vi "SQL_6220_data_insert.vi"(0 "数据":T1={"时间"=timestamp(3515985789.500352 s since 1904-01-01), "陪试轴承润滑单元出油温度1"=array[32000 elements], "陪试轴承润滑单元出油温度2"=array[32000 elements], "轴承外圈温度"=array[32000 elements], "出油温度"=array[32000 elements], "摩擦力1"=array[32000 elements], "摩擦力2"=array[32000 elements], "径向油缸力"=array[80000 elements], "轴向油缸力"=array[80000 elements], "转速"=array[80000 elements]}) -> (7 "error out":errorcluster, 8 "数据插入时间ms":u32)   [LabVIEW 2014]
uses:
  <vilib>/addons/database/Connection.llb/DB Tools Open Connec (String).vi
  <vilib>/addons/database/Connection.llb/Conn Execute.vi
  <vilib>/addons/database/Recordset.llb/Rec Destroy - Connection.vi
  <vilib>/addons/database/NI_Database_API.lvlib
panel:
  out "x-y":u32
  out "毫秒计时值 2":u32
  out "毫秒计时值":u32
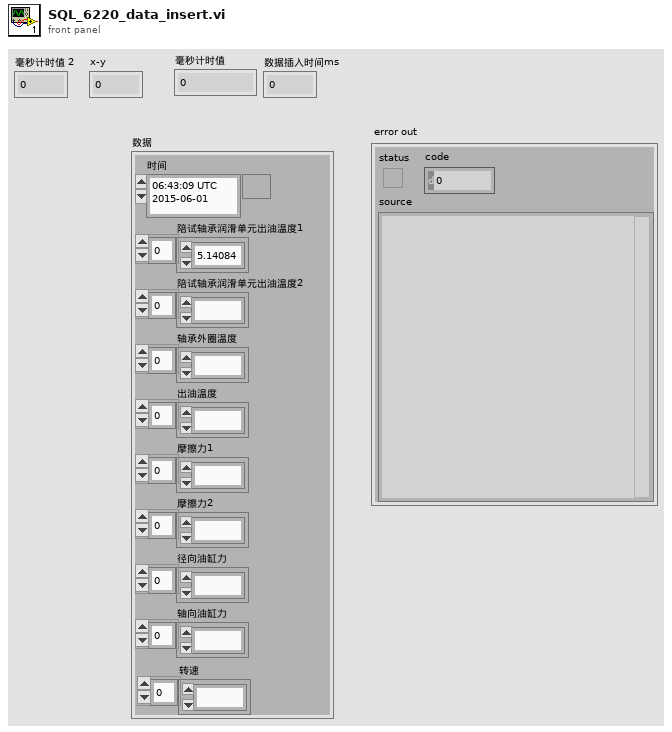
[diagram p1: front panel]
types:
  T1 = cluster{"时间":timestamp, "陪试轴承润滑单元出油温度1":sgl[], "陪试轴承润滑单元出油温度2":sgl[], "轴承外圈温度":sgl[], "出油温度":sgl[], "摩擦力1":sgl[], "摩擦力2":sgl[], "径向油缸力":sgl[], "轴向油缸力":sgl[], "转速":sgl[]}
  T2 = cluster{string, string, string, string, string, string, string, string, string}
  T3 = typedef "NI_Database_API.lvlib/Conn ObjectReference.ctl" = refnum<k1>
  T4 = typedef "NI_Database_API.lvlib/Rec ObjectReference.ctl" = refnum<k1>
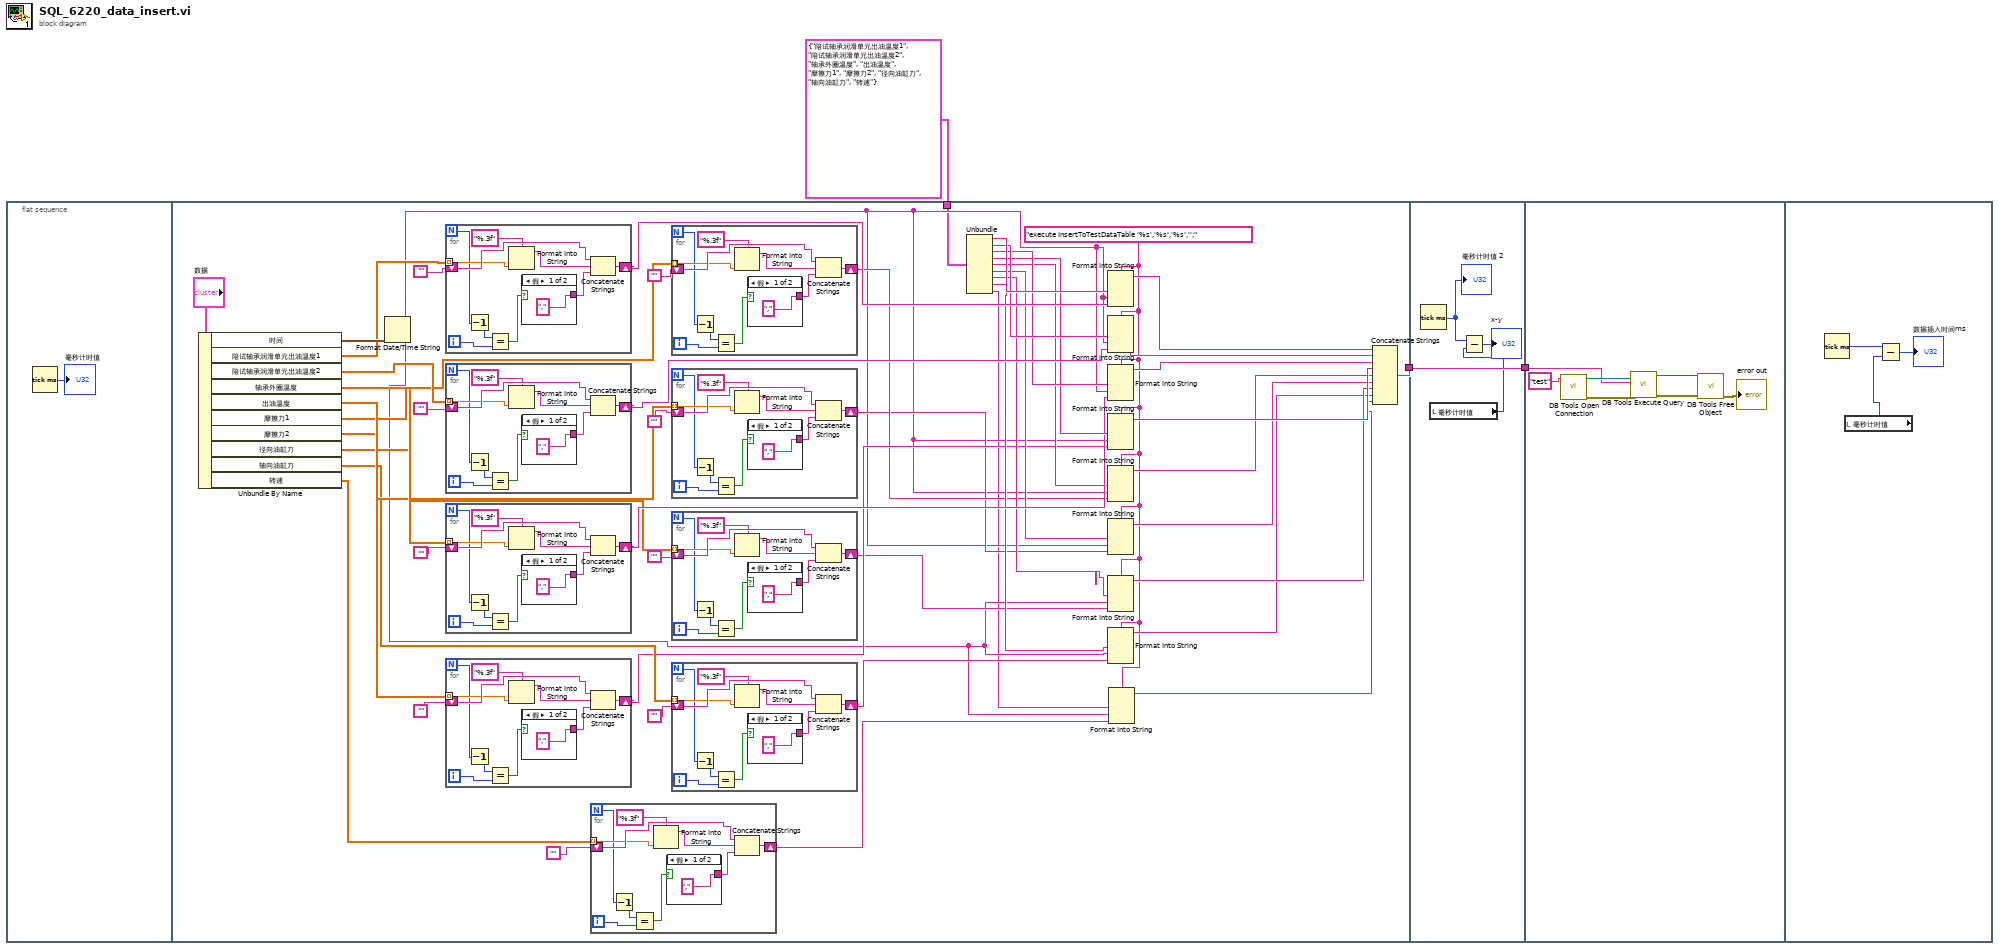
[diagram p0: block diagram]
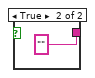
[diagram p2: hidden frame]
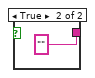
[diagram p3: hidden frame]
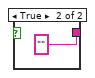
[diagram p4: hidden frame]
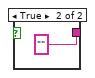
[diagram p5: hidden frame]
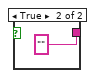
[diagram p6: hidden frame]
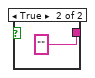
[diagram p7: hidden frame]
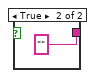
[diagram p8: hidden frame]
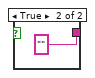
[diagram p9: hidden frame]
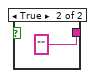
[diagram p10: hidden frame]
diagram:
  n1 = flat-sequence {
    tunnel: [w55] -> w3
    tunnel: T2 {"陪试轴承润滑单元出油温度1", "陪试轴承润滑单元出油温度2", "轴承外圈温度", "出油温度", "摩擦力1", "摩擦力2", "径向油缸力", "轴向油缸力", "转速"} ("通道名") -> [w5]
    tunnel: w3 -> [w167]
    tunnel: [w167] -> w2
    tunnel: w2 -> [w168]
    frame #0 {
      n2 = Tick Count (ms)() -> (millisecond timer value=→"毫秒计时值":u32)
    }
    frame #1 {
      w7 = "execute InsertToTestDataTable '%s','%s','%s','';"
      n3 = Unbundle By Name("数据") -> ("时间"=w54:timestamp, "陪试轴承润滑单元出油温度1"=w49:sgl[], "陪试轴承润滑单元出油温度2"=w48:sgl[], "轴承外圈温度"=w46:sgl[], "出油温度"=w44:sgl[], "摩擦力1"=w33:sgl[], "摩擦力2"=w32:sgl[], "径向油缸力"=w31:sgl[], "轴向油缸力"=w30:sgl[], "转速"=w12:sgl[])
      n4 = Format Date/Time String(seconds (now)=w54) -> (date/time string=w9:string)  [unwired: 2 in]
      n5 = for "For循环" {
        N -> [w154]
        tunnel: w49 -> [w159] mode=indexing
        shift-right: [w160] -> w51
        shift-left: "" -> [w161]
        i -> [w156]
        n6 = Decrement(x=w154) -> (x-1=w155:i32)
        n7 = Equal?(x=w155, y=w156) -> (x = y?=w153:bool)
        n8 = Format Into String(format string="%.3f", w159) -> (resulting string=w158:string)  [unwired: 2 in, 1 out]
        n9 = case shown="假" w153 {
          tunnel: ["," ""] -> w152
          frame False {
          }
          frame True {
          }
        }
        n10 = Concatenate Strings(w161, w158, w152) -> (w160:string)
      }
      n11 = for "For循环" {
        N -> [w142]
        tunnel: w48 -> [w147] mode=indexing
        shift-right: [w148] -> w42
        shift-left: "" -> [w149]
        i -> [w144]
        n12 = Decrement(x=w142) -> (x-1=w143:i32)
        n13 = Equal?(x=w143, y=w144) -> (x = y?=w141:bool)
        n14 = Format Into String(format string="%.3f", w147) -> (resulting string=w146:string)  [unwired: 2 in, 1 out]
        n15 = case shown="假" w141 {
          tunnel: ["," ""] -> w140
          frame False {
          }
          frame True {
          }
        }
        n16 = Concatenate Strings(w149, w146, w140) -> (w148:string)
      }
      n17 = for "For循环" {
        N -> [w130]
        tunnel: w46 -> [w135] mode=indexing
        shift-right: [w136] -> w37
        shift-left: "" -> [w137]
        i -> [w132]
        n18 = Decrement(x=w130) -> (x-1=w131:i32)
        n19 = Equal?(x=w131, y=w132) -> (x = y?=w129:bool)
        n20 = Format Into String(format string="%.3f", w135) -> (resulting string=w134:string)  [unwired: 2 in, 1 out]
        n21 = case shown="假" w129 {
          tunnel: ["," ""] -> w128
          frame False {
          }
          frame True {
          }
        }
        n22 = Concatenate Strings(w137, w134, w128) -> (w136:string)
      }
      n23 = for "For循环" {
        N -> [w118]
        tunnel: w44 -> [w123] mode=indexing
        shift-right: [w124] -> w21
        shift-left: "" -> [w125]
        i -> [w120]
        n24 = Decrement(x=w118) -> (x-1=w119:i32)
        n25 = Equal?(x=w119, y=w120) -> (x = y?=w117:bool)
        n26 = Format Into String(format string="%.3f", w123) -> (resulting string=w122:string)  [unwired: 2 in, 1 out]
        n27 = case shown="假" w117 {
          tunnel: ["," ""] -> w116
          frame False {
          }
          frame True {
          }
        }
        n28 = Concatenate Strings(w125, w122, w116) -> (w124:string)
      }
      n29 = for "For循环" {
        N -> [w58]
        tunnel: w12 -> [w63] mode=indexing
        shift-right: [w64] -> w10
        shift-left: "" -> [w65]
        i -> [w60]
        n30 = Decrement(x=w58) -> (x-1=w59:i32)
        n31 = Equal?(x=w59, y=w60) -> (x = y?=w57:bool)
        n32 = Format Into String(format string="%.3f", w63) -> (resulting string=w62:string)  [unwired: 2 in, 1 out]
        n33 = case shown="假" w57 {
          tunnel: ["," ""] -> w56
          frame False {
          }
          frame True {
          }
        }
        n34 = Concatenate Strings(w65, w62, w56) -> (w64:string)
      }
      n35 = for "For循环" {
        N -> [w106]
        tunnel: w33 -> [w111] mode=indexing
        shift-right: [w112] -> w20
        shift-left: "" -> [w113]
        i -> [w108]
        n36 = Decrement(x=w106) -> (x-1=w107:i32)
        n37 = Equal?(x=w107, y=w108) -> (x = y?=w105:bool)
        n38 = Format Into String(format string="%.3f", w111) -> (resulting string=w110:string)  [unwired: 2 in, 1 out]
        n39 = case shown="假" w105 {
          tunnel: ["," ""] -> w104
          frame False {
          }
          frame True {
          }
        }
        n40 = Concatenate Strings(w113, w110, w104) -> (w112:string)
      }
      n41 = for "For循环" {
        N -> [w94]
        tunnel: w32 -> [w99] mode=indexing
        shift-right: [w100] -> w19
        shift-left: "" -> [w101]
        i -> [w96]
        n42 = Decrement(x=w94) -> (x-1=w95:i32)
        n43 = Equal?(x=w95, y=w96) -> (x = y?=w93:bool)
        n44 = Format Into String(format string="%.3f", w99) -> (resulting string=w98:string)  [unwired: 2 in, 1 out]
        n45 = case shown="假" w93 {
          tunnel: ["," ""] -> w92
          frame False {
          }
          frame True {
          }
        }
        n46 = Concatenate Strings(w101, w98, w92) -> (w100:string)
      }
      n47 = for "For循环" {
        N -> [w82]
        tunnel: w31 -> [w87] mode=indexing
        shift-right: [w88] -> w18
        shift-left: "" -> [w89]
        i -> [w84]
        n48 = Decrement(x=w82) -> (x-1=w83:i32)
        n49 = Equal?(x=w83, y=w84) -> (x = y?=w81:bool)
        n50 = Format Into String(format string="%.3f", w87) -> (resulting string=w86:string)  [unwired: 2 in, 1 out]
        n51 = case shown="假" w81 {
          tunnel: ["," ""] -> w80
          frame False {
          }
          frame True {
          }
        }
        n52 = Concatenate Strings(w89, w86, w80) -> (w88:string)
      }
      n53 = for "For循环" {
        N -> [w70]
        tunnel: w30 -> [w75] mode=indexing
        shift-right: [w76] -> w17
        shift-left: "" -> [w77]
        i -> [w72]
        n54 = Decrement(x=w70) -> (x-1=w71:i32)
        n55 = Equal?(x=w71, y=w72) -> (x = y?=w69:bool)
        n56 = Format Into String(format string="%.3f", w75) -> (resulting string=w74:string)  [unwired: 2 in, 1 out]
        n57 = case shown="假" w69 {
          tunnel: ["," ""] -> w68
          frame False {
          }
          frame True {
          }
        }
        n58 = Concatenate Strings(w77, w74, w68) -> (w76:string)
      }
      n59 = Unbundle(w5) -> (w41:string, w40:string, w39:string, w38:string, w25:string, w24:string, w23:string, w22:string, w8:string)
      n60 = Format Into String ("格式化写入字符串")(format string=w7, w41, w9, w51) -> (resulting string=w53:string)  [unwired: 2 in, 1 out]
      n61 = Format Into String ("格式化写入字符串")(format string=w7, w40, w9, w42) -> (resulting string=w36:string)  [unwired: 2 in, 1 out]
      n62 = Format Into String ("格式化写入字符串")(format string=w7, w39, w9, w37) -> (resulting string=w35:string)  [unwired: 2 in, 1 out]
      n63 = Format Into String ("格式化写入字符串")(format string=w7, w38, w9, w21) -> (resulting string=w34:string)  [unwired: 2 in, 1 out]
      n64 = Format Into String ("格式化写入字符串")(format string=w7, w25, w9, w20) -> (resulting string=w16:string)  [unwired: 2 in, 1 out]
      n65 = Format Into String ("格式化写入字符串")(format string=w7, w24, w9, w19) -> (resulting string=w15:string)  [unwired: 2 in, 1 out]
      n66 = Format Into String ("格式化写入字符串")(format string=w7, w23, w9, w18) -> (resulting string=w14:string)  [unwired: 2 in, 1 out]
      n67 = Format Into String ("格式化写入字符串")(format string=w7, w22, w9, w17) -> (resulting string=w13:string)  [unwired: 2 in, 1 out]
      n68 = Format Into String ("格式化写入字符串")(format string=w7, w8, w9, w10) -> (resulting string=w6:string)  [unwired: 2 in, 1 out]
      n69 = Concatenate Strings ("连接字符串")(w53, w36, w35, w34, w16, w15, w14, w13, w6) -> (w55:string)
    }
    frame #2 {
      n70 = Tick Count (ms)() -> (millisecond timer value=w166:u32)
      "毫秒计时值 2" <- w166
      n71 = local read "毫秒计时值"() -> (w165:u32)
      n72 = Subtract(x=w166, y=w165) -> (x-y=→"x-y":u32)
    }
    frame #3 {
      n73 = call-poly <vilib>:"DB Tools Open Connection.vi"("connection information"="test") -> ("error out"=w174:errorcluster, "connection reference"=w173:T3)  [unwired: 7 in]
      n74 = call-poly <vilib>:"DB Tools Execute Query.vi"("error in (no error)"=w174, "SQL query"=w168, "connection reference"=w173) -> ("error out"=w171:errorcluster, "recordset reference"=w170:T4)  [unwired: 5 in]
      n75 = call-poly <vilib>:"DB Tools Free Object.vi"("error in (no error)"=w171, "recordset reference"=w170) -> ("error out"=→"error out":errorcluster)  [unwired: 8 in, 1 out]
    }
    frame #4 {
      n76 = Tick Count (ms)() -> (millisecond timer value=w177:u32)
      n77 = local read "毫秒计时值"() -> (w175:u32)
      n78 = Subtract(x=w177, y=w175) -> (x-y=→"数据插入时间ms":u32)
    }
  }
